vi "Write_FreqSweep_Impedance_Meas.vi"(0 "Meta-Data Array":dbl[](array[numeric])=[1.0], 4 "Z_Phase_Vec":dbl[](array[numeric]), 5 "Freq Vector":dbl[](array[numeric]), 6 "|Z| Vector":dbl[](array[numeric]), 7 "Compensation and Gain":T1={"Rg_Vmon"=5000.0, "Rg_Imon"=5000.0, "ESL_Cal"=2.5e-07, "ESR_Cal"=0.0, "Cp_Cal"=0.0, "Rp_Cal"=0.0, "Use Open/Short\nCompensation"=FALSE, "R_Shunt"=10000.0, "RLoad"=1000000000.0, "RLoad_Meas"=1000000000.0} {"RLoad_Meas" format="%#_6p"; "RLoad" format="%#_6p"}, 8 "Test Params Cluster":T2={"Test Freq. (Hz)"=0.0, "Output Signal Amplitude\nVolts Pk"=0.0, "Sampling Time (s)"=0.0, "Sampling Rate (Hz)"=0.0, "Output Channel"="Dev2/ao0", "Current Channel"="Dev2/ai0", "Voltage Channel"="Dev2/ai0", "Trigger Channel"="/Dev2/ao/StartTrigger", "Number of runs"=5}, 9 "Experiment Title":string="Experiment Title", 10 "File Name String":string="Test", 11 "Path":path=path "C:/Users/MPI/Documents/Test Saving Data") -> ()   [LabVIEW 2022 SP3]
panel:
  out "TDMS path":path=path "C:/Users/MPI/Documents/Test Saving Data/2022_01_06_23_07_06_Test.tdms"
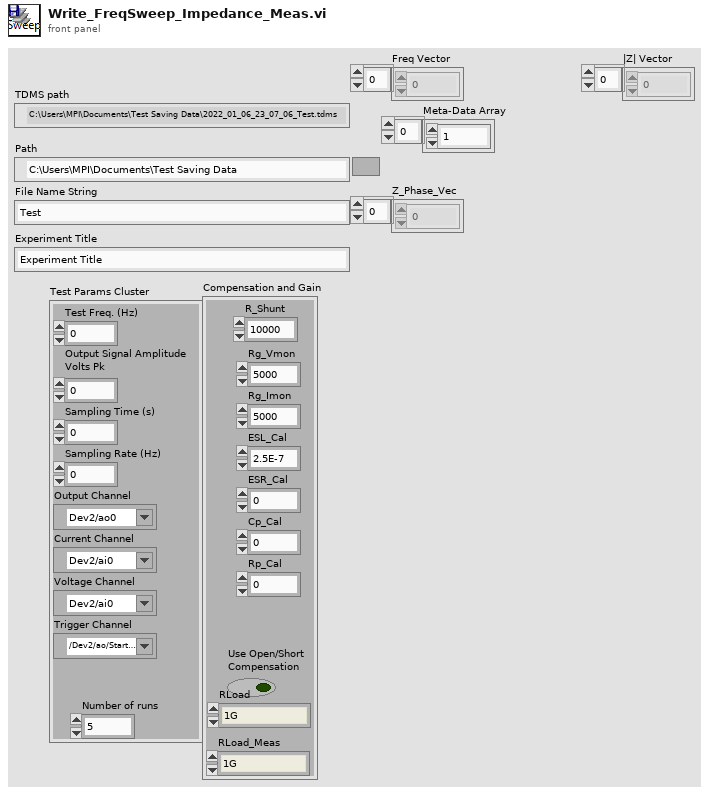
[diagram p1: front panel]
types:
  T1 = cluster{"Rg_Vmon":dbl, "Rg_Imon":dbl, "ESL_Cal":dbl, "ESR_Cal":dbl, "Cp_Cal":dbl, "Rp_Cal":dbl, "Use Open/Short\nCompensation":bool, "R_Shunt":dbl, "RLoad":dbl, "RLoad_Meas":dbl}
  T2 = cluster{"Test Freq. (Hz)":dbl, "Output Signal Amplitude\nVolts Pk":dbl, "Sampling Time (s)":dbl, "Sampling Rate (Hz)":dbl, "Output Channel":tag, "Current Channel":tag, "Voltage Channel":tag, "Trigger Channel":tag, "Number of runs":i32}
  T3 = enum16{"open", "open or create", "create or replace", "create", "open (read-only)"}
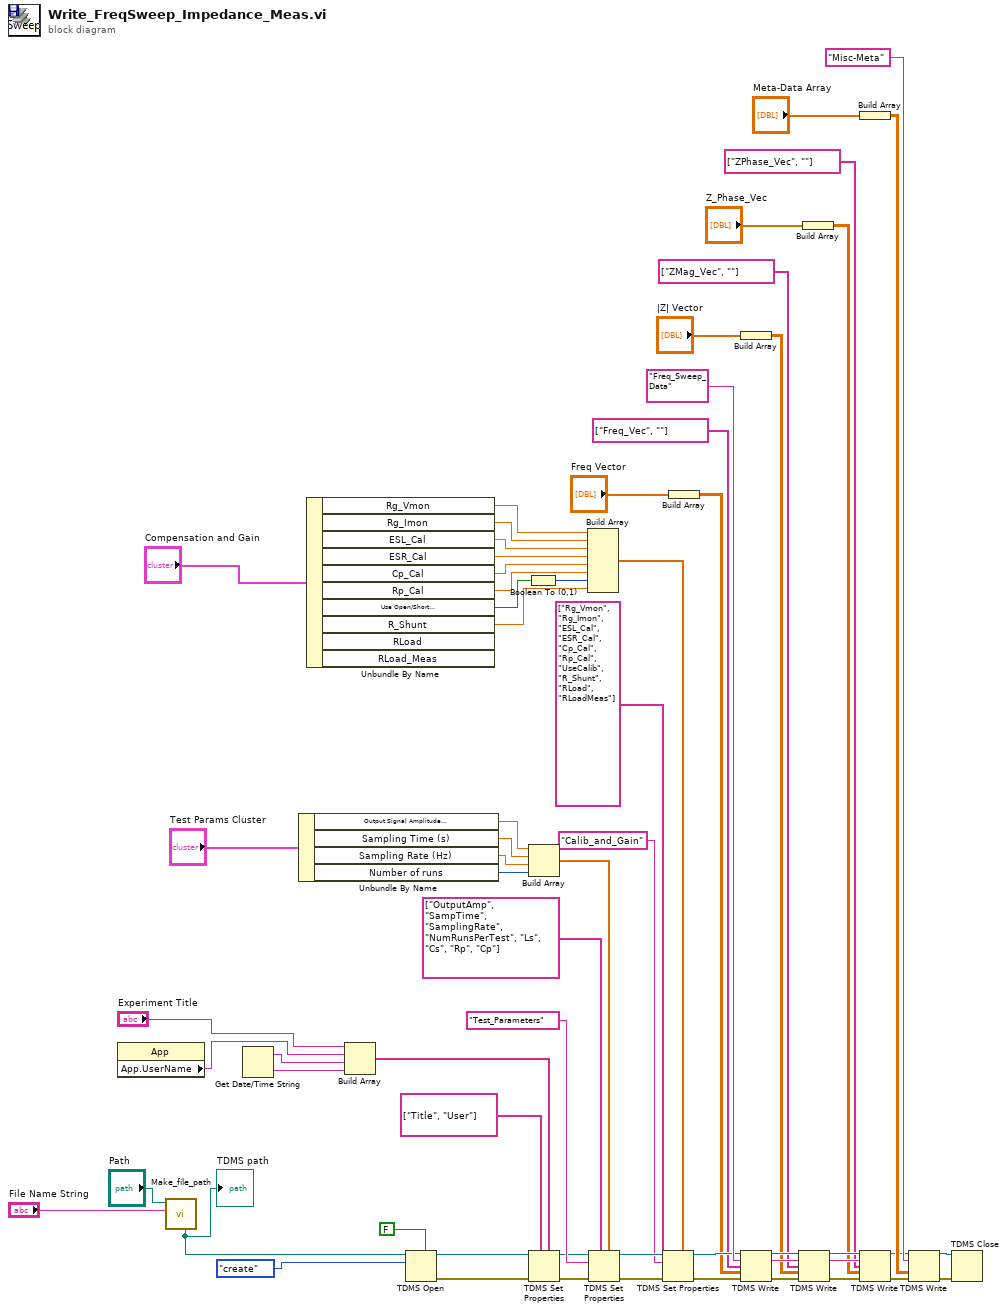
[diagram p0: block diagram]
diagram:
  n1 = property class="App"() -> ("App.UserName"=w58:string)  [unwired: 2 in, 2 out]
  n2 = call "Make_file_path.vi"("File Name String"="File Name String", "Base path"="Path") -> ("TDMS path"=w63:path)  [unwired: 9 in]
  "TDMS path" <- w63
  n3 = Get Date/Time String() -> (date string=w54:string, time string=w53:string)  [unwired: 3 in]
  n4 = Unbundle By Name("Test Params Cluster") -> ("Output Signal Amplitude\nVolts Pk"=w46:dbl, "Sampling Time (s)"=w47:dbl, "Sampling Rate (Hz)"=w48:dbl, "Number of runs"=w8:i32)
  n5 = Unbundle By Name("Compensation and Gain") -> ("Rg_Vmon"=w38:dbl, "Rg_Imon"=w37:dbl, "ESL_Cal"=w36:dbl, "ESR_Cal"=w35:dbl, "Cp_Cal"=w34:dbl, "Rp_Cal"=w33:dbl, "Use Open/Short\nCompensation"=w32:bool, "R_Shunt"=w29:dbl)  [unwired: 2 out]
  n6 = Build Array("Experiment Title", w58, w54, w53) -> (w57:string[])
  n7 = TDMS Open(5:FALSE ("create index file? (T)"), 10:T3."create" ("operation (0:open)"), 11:w63) -> (0:w52:errorcluster, 3:w55:refnum<k34>)  [unwired: 4 in]
  n8 = Boolean To (0,1)(Boolean=w32) -> (0, 1=w31:i16)
  n9 = Build Array(w46, w47, w48, w8) -> (w45:dbl[])
  n10 = TDMS Set Properties(5:w57, 7:string[] ["Title", "User"] ("property names"), 8:w52, 11:w55) -> (0:w27:errorcluster, 3:w28:refnum<k34>)  [unwired: 4 out]
  n11 = Build Array(w38, w37, w36, w35, w34, w33, w31, w29) -> (w30:dbl[])
  n12 = TDMS Set Properties(5:w45, 7:string[] ["OutputAmp", "SampTime", "SamplingRate", "NumRunsPerTest", "Ls", "Cs", "Rp", "Cp"] ("property names"), 8:w27, 10:"Test_Parameters" ("group name"), 11:w28) -> (0:w41:errorcluster, 3:w42:refnum<k34>)  [unwired: 3 out]
  n13 = TDMS Set Properties(5:w30, 7:string[] ["Rg_Vmon", "Rg_Imon", "ESL_Cal", "ESR_Cal", "Cp_Cal", "Rp_Cal", "UseCalib", "R_Shunt", "RLoad", "RLoadMeas"] ("property names"), 8:w41, 10:"Calib_and_Gain" ("group name"), 11:w42) -> (0:w18:errorcluster, 3:w19:refnum<k34>)  [unwired: 3 out]
  n14 = Build Array("Freq Vector") -> (w12:dbl[][])
  n15 = Build Array("|Z| Vector") -> (w15:dbl[][])
  n16 = TDMS Write(0:w19, 5:"Freq_Sweep_Data" ("group name"), 7:string[] ["Freq_Vec", ""] ("property names"), 9:w12, 11:w18) -> (4:w22:refnum<k34>, 6:w21:string, 15:w23:errorcluster)  [unwired: 1 in, 1 out]
  n17 = TDMS Write(0:w22, 5:w21, 7:string[] ["ZMag_Vec", ""] ("property names"), 9:w15, 11:w23) -> (4:w25:refnum<k34>, 6:w24:string, 15:w26:errorcluster)  [unwired: 1 in, 1 out]
  n18 = Build Array("Z_Phase_Vec") -> (w17:dbl[][])
  n19 = Build Array("Meta-Data Array") -> (w5:dbl[][])
  n20 = TDMS Write(0:w25, 5:w24, 7:string[] ["ZPhase_Vec", ""] ("property names"), 9:w17, 11:w26) -> (4:w1:refnum<k34>, 15:w4:errorcluster)  [unwired: 1 in, 2 out]
  n21 = TDMS Write(0:w1, 5:"Misc-Meta" ("group name in (Untitled)"), 9:w5, 11:w4) -> (4:w2:refnum<k34>, 15:w3:errorcluster)  [unwired: 2 in, 2 out]
  n22 = TDMS Close(8:w3, 11:w2) -> ()  [unwired: 2 out]
